vi "nominal user me.vi"(8 "error in (no error)":errorcluster, 10 "out_user":i32, 11 "client":i32) -> (0 "error out":errorcluster, 2 "out_user out":i32, 3 "function return":i32)   [LabVIEW 2020, in "client.lvlib"]
doc: "int32_t nominal_user_me(int32_t client, int32_t *out_user);"
uses:
  client.lvlib
  bin/nominalClient_64.dll
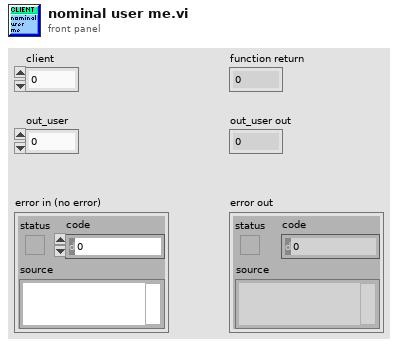
[diagram p1: front panel]
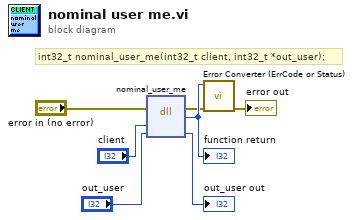
[diagram p0: block diagram]
diagram:
  # "int32_t nominal_user_me(int32_t client, int32_t *out_user);"
  n1 = dll-call lib="C:/code/labview-client-rs/lv_src/bin/nominalClient_*.*" fn="nominal_user_me"(error in="error in (no error)", "client"="client", "out_user"="out_user") -> (error out=w2:errorcluster, w7:i32, "out_user"=→"out_user out":i32)  [unwired: 3 in, 1 out]
  "function return" <- w7
  n2 = call "Error Converter (ErrCode or Status).vi"("error in (no error)"=w2, "error code"=w7) -> ("error out"=→"error out":errorcluster)  [unwired: 9 in]
